vi "GetAxisParameterDouble.vi"(8 "error in (no error)":errorcluster, 9 "Parameter Name":string(combo), 10 "axis name":string, 11 "controller in":refnum<k24>) -> (0 "error out":errorcluster, 2 "value":dbl, 3 "controller out":refnum<k24>)   [LabVIEW 2019, in "Aerotech VIs.lvlib"]
uses:
  C:/Program Files (x86)/Aerotech/A3200/LabVIEW/2010/Bin/Aerotech.A3200.dll
  Program Files (x86)/Aerotech/A3200/LabVIEW/2010/Bin/Aerotech.A3200.dll
  C:/Users/HEP/Documents/Aerotech gantry/V5/UCSB-Gantry-master/V5/Drivers/Aerotech A3200/Bin/Aerotech.A3200.LabVIEW.dll
  Bin/Aerotech.A3200.LabVIEW.dll
  Aerotech VIs.lvlib
panel:
  out "ParameterType":i32(ring)=1 items=["Integer", "Double", "Single", "Long", "String"]
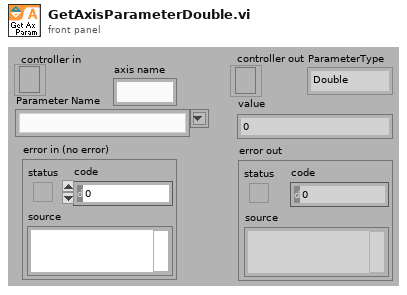
[diagram p1: front panel]
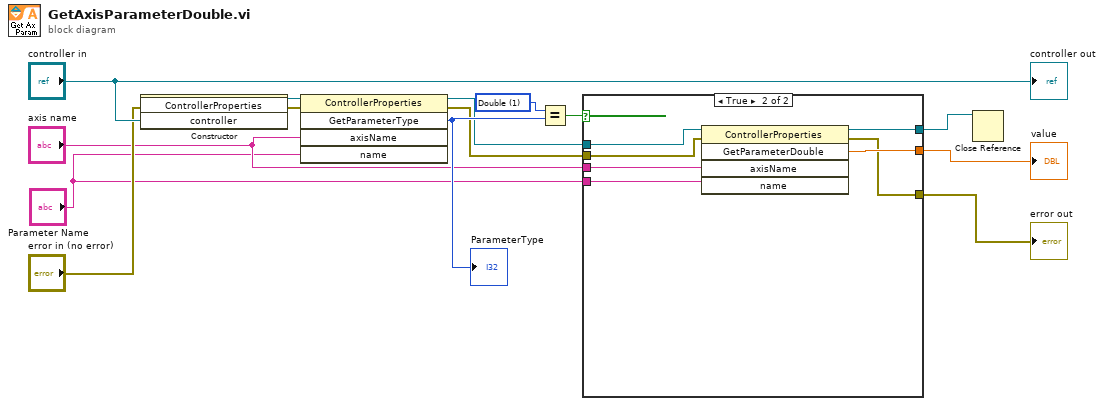
[diagram p0: block diagram]
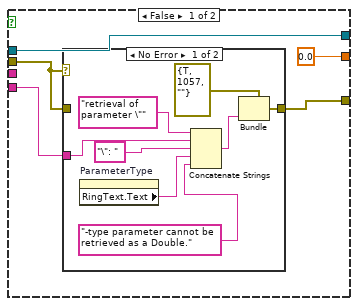
[diagram p2: hidden frame]
diagram:
  w10 = 1 items=["Integer", "Double", "Single", "Long", "String"] ("GetParameterType")
  n1 = constructor class="ControllerProperties"(error in="error in (no error)", "controller"="controller in") -> (reference out=w12:refnum<k24>, error out=w11:errorcluster)  [unwired: 2 in, 2 out]
  n2 = invoke class="ControllerProperties" method="GetParameterType"(reference=w12, error in=w11, "axisName"="axis name", "name"="Parameter Name") -> (reference out=w6:refnum<k24>, error out=w5:errorcluster, "GetParameterType"=w9:i32)  [unwired: 1 in, 2 out]
  "ParameterType" <- w9
  n3 = Equal?(x=w10, y=w9) -> (x = y?=w8:bool)
  n4 = case shown="True" w8 {
    tunnel: [w19 w34] -> w7
    tunnel: w6 -> [w19 w35]
    tunnel: "Parameter Name" -> [w15 w30]
    tunnel: w5 -> [w16 w33]
    tunnel: [0.0 w32] -> w4
    tunnel: [w17 w31] -> w3
    tunnel: "axis name" -> [_ w29]
    frame False {
      n5 = case shown="No Error" w16 {
        tunnel: [w26 w28] -> w17
        tunnel: w16 -> [_ w28]
        tunnel: w15 -> [w23 _]
        frame No Error {
          n6 = property on="ParameterType" class="Ring (strict)"() -> ("RingText.Text"=w21:string)  [unwired: 2 in, 2 out]
          n7 = Concatenate Strings("retrieval of parameter \"" ("string"), w23, "\": " ("string"), w21, "-type parameter cannot be retrieved as a Double." ("string")) -> (w25:string)
          n8 = Bundle(cluster=cluster{bool, "code":i32, "source":string} {TRUE, "code"=1057, "source"=""} ("error out"), "source"=w25) -> (w26:cluster{bool, "code":i32, "source":string})  [unwired: 2 in]
        }
        frame Error {
        }
      }
    }
    frame True {
      n9 = invoke class="ControllerProperties" method="GetParameterDouble"(reference=w35, error in=w33, "axisName"=w29, "name"=w30) -> (reference out=w34:refnum<k24>, error out=w31:errorcluster, "GetParameterDouble"=w32:dbl)  [unwired: 1 in, 2 out]
    }
  }
  "error out" <- w3
  "value" <- w4
  n10 = Close Reference(reference=w7) -> ()  [unwired: 1 in, 1 out]
  "controller out" <- "controller in"
